vi "photo_encoder_new2.vi"() -> ()   [LabVIEW 2014]
panel:
  out "Marks/second":dbl
  out "Marks":dbl
  in  "Brightness of Mark":dbl
  in  "Photo Value(placeholder for sensor data)":dbl
  # "This VI recognizes significant increases in brightness as \"marks\" and outputs the number of marks detected in the last second.\nKnown issues:  Does not reset M/s consistently, just like photo_encoder_new.  Turning a section into a subVI doesn't seem to help."
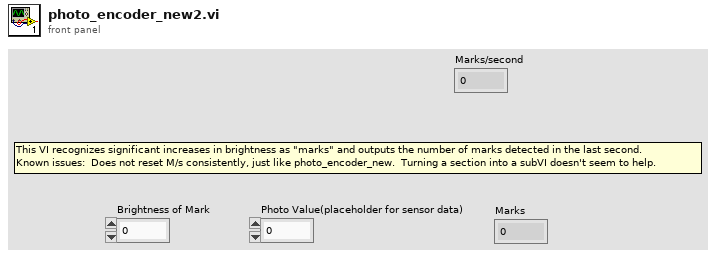
[diagram p1: front panel]
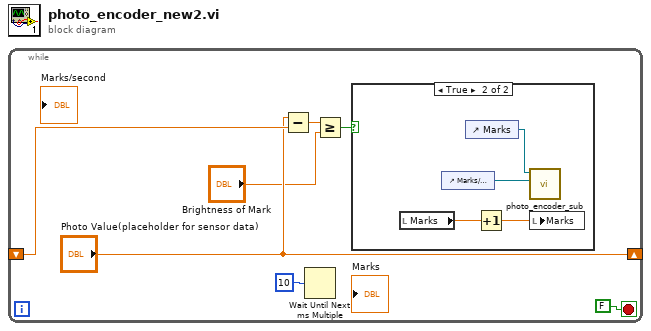
[diagram p0: block diagram]
diagram:
  n1 = while {
    shift-right: ["Photo Value(placeholder for sensor data)"] -> _
    shift-left: _ -> [w7]
    stop <- FALSE stop-if-true
    n2 = Subtract(x="Photo Value(placeholder for sensor data)", y=w7) -> (x-y=w5:dbl)
    n3 = Wait Until Next ms Multiple(millisecond multiple=u32 10) -> ()  [unwired: 1 out]
    n4 = Greater Or Equal?(x=w5, y="Brightness of Mark") -> (x >= y?=w3:bool)
    n5 = case shown="True" w3 {
      frame False {
      }
      frame True {
        n6 = local read "Marks"() -> (w10:dbl)
        n7 = control-ref of="Marks/second"() -> (w8:refnum<vi>)
        n8 = control-ref of="Marks"() -> (w9:refnum<vi>)
        n9 = Increment(x=w10) -> (x+1=w11:dbl)
        n10 = call "photo_encoder_sub.vi"("reference"=w8, "Digital in"=w9) -> ()  [unwired: 10 in]
        n11 = local write "Marks"(w11) -> ()
      }
    }
  }
